vi "数据库全局.vi"() -> ()   [LabVIEW 2017]
panel:
  in  "database路径":path=path "D:/database.db"
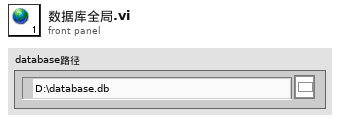
[diagram p1: front panel]
diagram:
